vi "Close.vi"(8 "error in":errorcluster, 11 "Power Nominal Value in":refnum<class "Power Nominal Value.lvclass">) -> (0 "error out":errorcluster, 3 "Power Nominal Value out":refnum<class "Power Nominal Value.lvclass">)   [LabVIEW 2023, in "Power Nominal Value.lvclass"]
uses:
  Power Nominal Value.lvclass
  Parents/Nominal Value/Nominal Value.lvclass
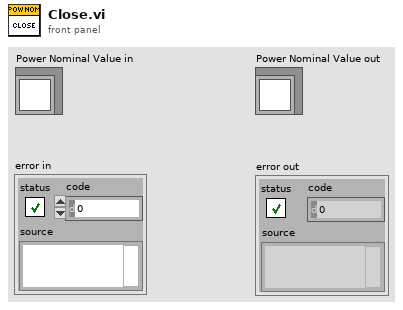
[diagram p1: front panel]
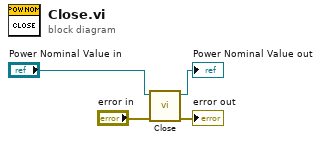
[diagram p0: block diagram]
diagram:
  n1 = call-parent "Close.vi"("error in"="error in", "Nominal Value in"="Power Nominal Value in") -> ("error out"=→"error out":errorcluster, "Nominal Value out"=→"Power Nominal Value out":refnum<class "Power Nominal Value.lvclass">)  [unwired: 8 in]
